vi "MatLab.vi"(2 "Segment":dbl, 3 "input Array":dbl[](array[numeric]), 4 "Levels":dbl=5.0, 5 "WaveletType":string="db04") -> (0 "Detected Wave":string, 1 "dominantFrequency":dbl)   [LabVIEW 2023]
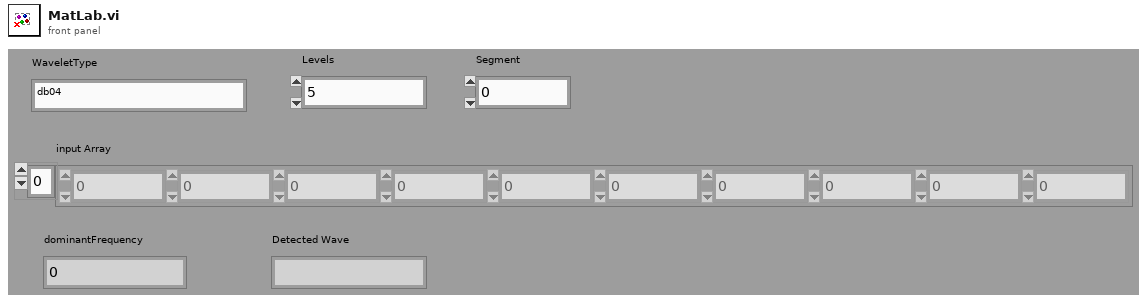
[diagram p1: front panel]
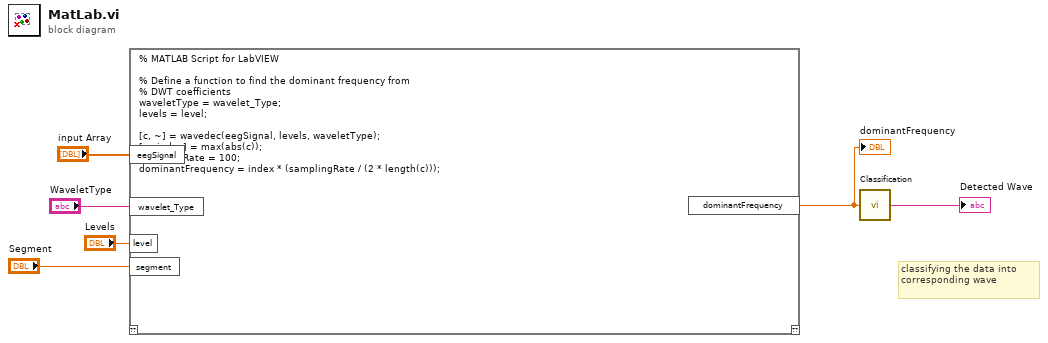
[diagram p0: block diagram]
diagram:
  # "classifying the data into\ncorresponding wave"
  n1 = script code="% MATLAB Script for LabVIEW\n\n% Define a function to find the dominant frequency from\n% DWT coefficients\nwaveletType = wavelet_Type;\nlevels = level;\n\n[c, ~] = wavedec(eegSignal, levels, waveletType);\n[~, index] = max(abs(c));\nsamplingRate = 100;\ndominantFrequency = index * (samplingRate / (2 * length(c)));"("eegSignal"="input Array", "wavelet_Type"="WaveletType", "level"="Levels", "segment"="Segment") -> ("dominantFrequency"=w3:dbl)  [unwired: 1 in, 1 out]
  "dominantFrequency" <- w3
  n2 = call "Classification.vi"("Numeric"=w3) -> ("Detected Wave"=→"Detected Wave":string)
